vi "Lin Daten laden speichern.vi"(6 "Stufen Tabelle":T1, 9 "Lin Daten":T2 {"CalGas Eingang" items=["Cal Gas 1", "Cal Gas 2", "Cal Gas 3"]; "Max Fehler (Sollwert)" format="%#_5g"; "Zeitdauer Stufe" format="%#_5g"; "Anzahl Stufen" format="%#_5g"; "Verdünnungsgas" items=["N2", "O2"]}, 11 "Aktionen":T6) -> (0 "Stufen Tabellen":T1, 1 "Lin Daten Array":T2 {"CalGas Eingang" items=["Cal Gas 1", "Cal Gas 2", "Cal Gas 3"]; "Max Fehler (Sollwert)" format="%#_5g"; "Zeitdauer Stufe" format="%#_5g"; "Anzahl Stufen" format="%#_5g"; "Verdünnungsgas" items=["N2", "O2"]}, 3 "Gefunden?":bool)   [LabVIEW 2020, in "Linearisierung v2.lvlib" / "Gasteiler.lvlib"]
uses:
  Gasteiler.lvlib
  Lin Daten.ctl
  Visualisierungs Elemente/String - Eingabefeld.ctl
  Visualisierungs Elemente/Zahlen-Eingabefeld.ctl
  Lin Daten verwalten Aktionen.ctl
  Stufen Tabelle.ctl
  Seiten/FT-IR/FGV FT-IR Gasliste Aktionen.ctl
  Messdaten/Aktionen FGV Messdaten.ctl
  <vilib>/Utility/config.llb/Write Key (String).vi
  <vilib>/Utility/config.llb/Write Key (U32).vi
  <vilib>/Utility/config.llb/Write Key (Double).vi
  <vilib>/Utility/config.llb/Read Key (Double).vi
  <vilib>/Utility/config.llb/Read Key (U32).vi
  <vilib>/Utility/config.llb/Read Key (String).vi
  <vilib>/Utility/config.llb/NI_LVConfig.lvlib
  Allgemein/allgemeine Sub-VIs.lvlib
  Seiten/FT-IR/FT-IR.lvlib
  Messdaten/Messdaten.lvlib
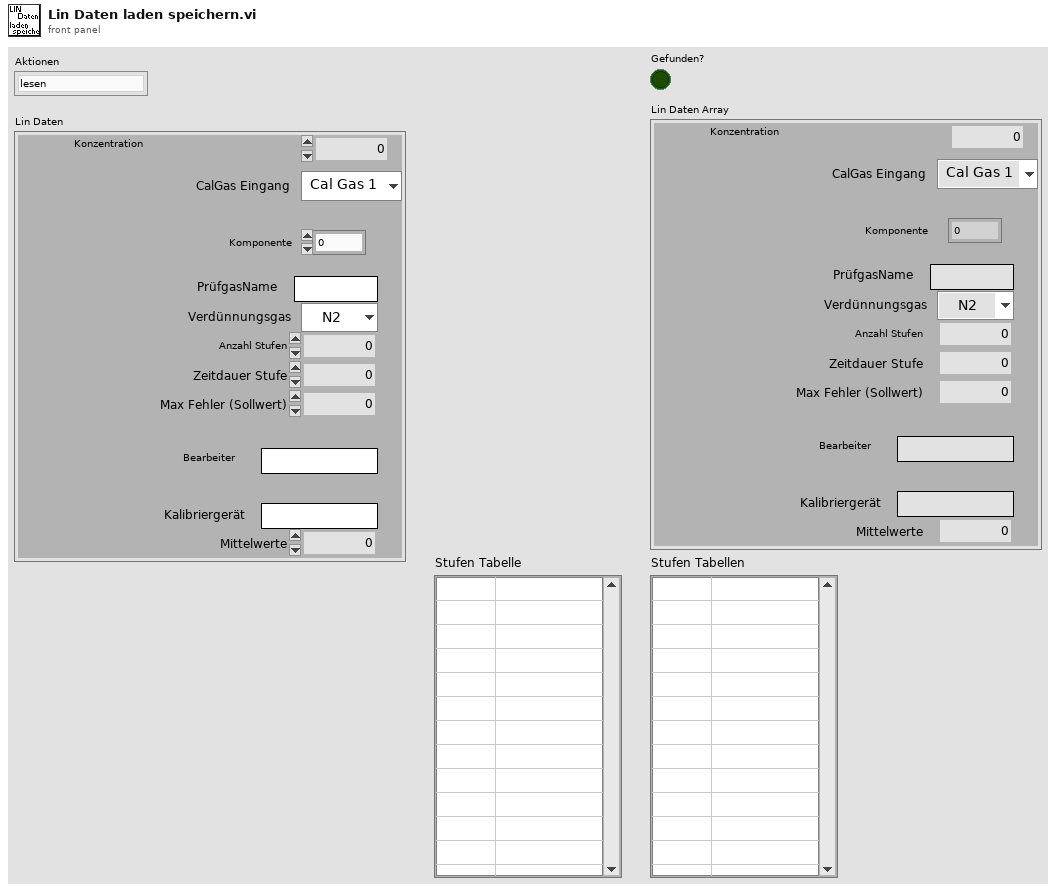
[diagram p1: front panel]
types:
  T1 = typedef "Linearisierung v2.lvlib/Gasteiler.lvlib/Stufen Tabelle.ctl" = string[][]
  T2 = typedef "Linearisierung v2.lvlib/Gasteiler.lvlib/Lin Daten.ctl" = cluster{"PrüfgasName":T3, "Verdünnungsgas":T4, "Anzahl Stufen":T5, "Zeitdauer Stufe":T5, "Max Fehler (Sollwert)":T5, "Bearbeiter":T3, "Kalibriergerät":T3, "Mittelwerte":i32, "Komponente":u16, "CalGas Eingang":u16, "Konzentration":sgl}
  T3 = typedef "String - Eingabefeld.ctl" = string
  T4 = typedef "Linearisierung v2.lvlib/Gasteiler.lvlib/Prüfgas in.ctl" = u16
  T5 = typedef "Zahlen-Eingabefeld.ctl" = sgl
  T6 = typedef "Linearisierung v2.lvlib/Gasteiler.lvlib/Lin Daten verwalten Aktionen.ctl" = enum16{"lesen", "speichern", "laden", "Lin Daten schr.", "Stufen Tabelle", "Lin Name AK", "Lin Pfad AK", "Umkehren"}
  T7 = typedef "Messdaten.lvlib/Aktionen FGV Messdaten.ctl" = enum16{"lesen", "schreiben", "löschen", "Mittelwerte", "Komponente"}
  T8 = typedef "FT-IR.lvlib/FGV FT-IR Gasliste Aktionen.ctl" = enum16{"lesen", "Gasliste FT-IR", "Gasliste ausgelesen", "laden", "speichern", "löschen"}
  T9 = typedef "String - Ausgabefeld.ctl" = string
  T10 = typedef "NI_LVConfig.lvlib/Config Data RefNum.ctl" = refnum<k1>
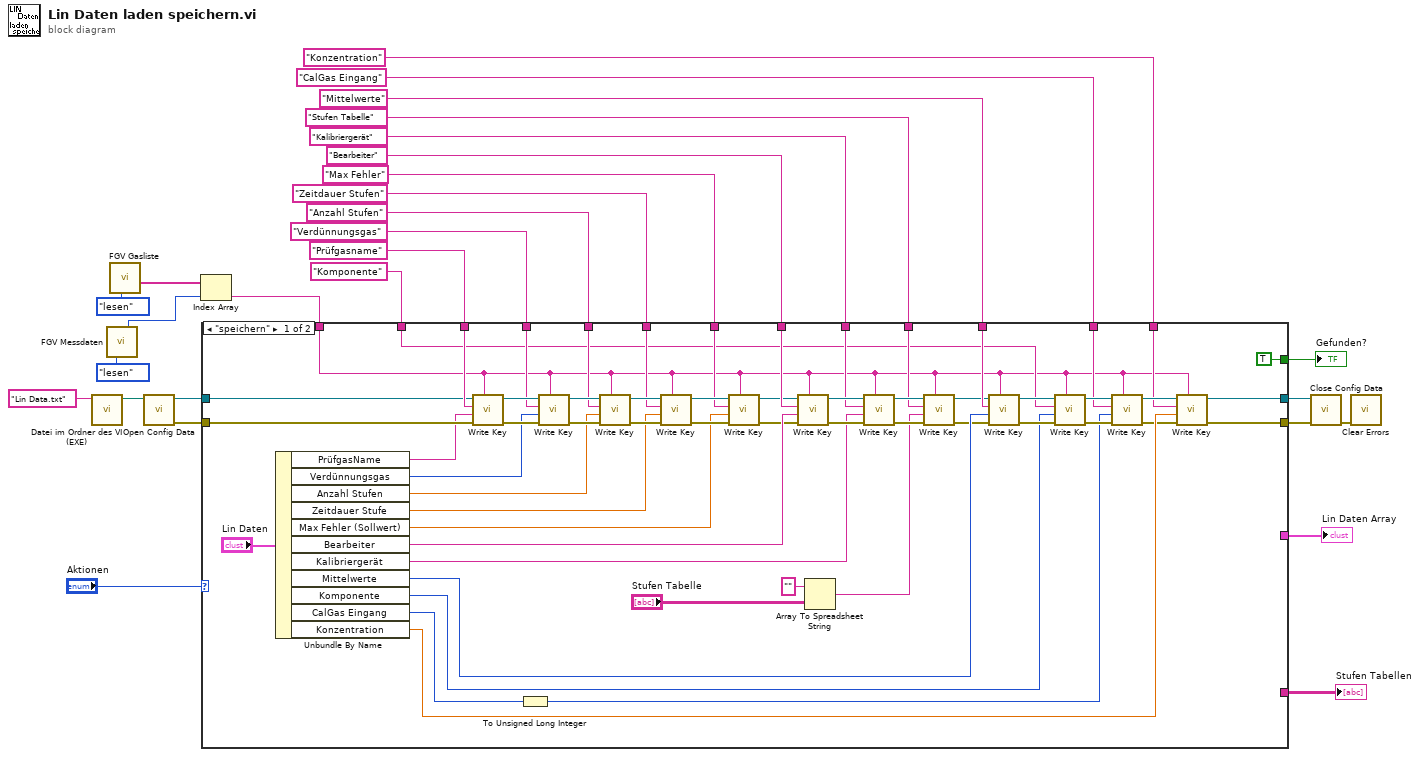
[diagram p0: block diagram]
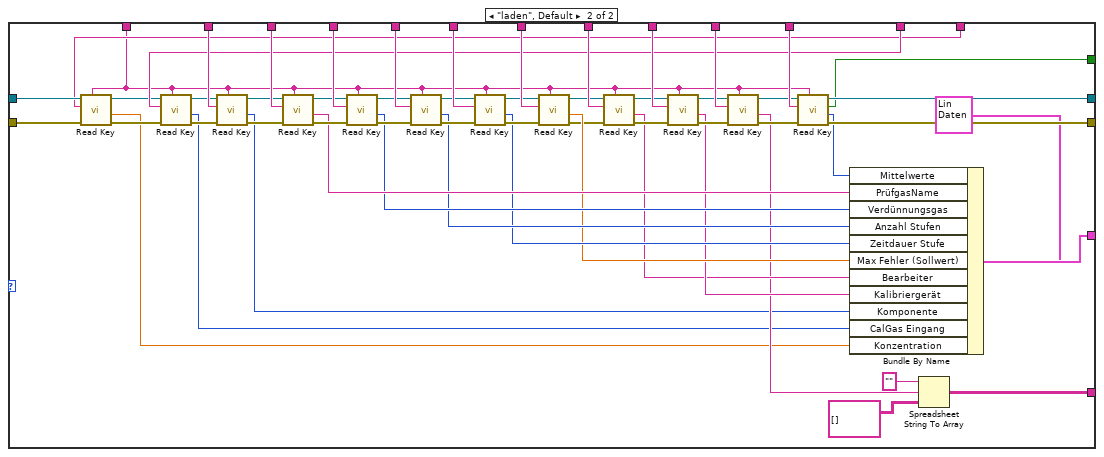
[diagram p2: hidden frame]
diagram:
  n1 = call "Datei im Ordner des VI (EXE).vi"("Dateiname"="Lin Data.txt") -> ("Dateipfad im Ordner des Haupt-VIs"=w28:path)  [unwired: 8 in, 2 out]
  n2 = call "FGV Messdaten.vi"("Aktionen"=Aktionen_FGV_Messdaten."lesen") -> ("Komponente"=w6:u16)  [unwired: 6 in, 8 out]
  n3 = call "FGV Gasliste.vi"("Aktionen"=FGV_FT-IR_Gasliste_Aktionen."lesen") -> ("Aktuelle Gasliste gesamt"=w4:T9[])  [unwired: 8 in, 2 out]
  n4 = call <vilib>:"Open Config Data.vi"("configuration file path"=w28) -> ("error out"=w25:errorcluster, "refnum"=w26:T10)  [unwired: 8 in, 1 out]
  n5 = Index Array(array=w4, index=w6) -> (element=w2:T9)
  n6 = case shown="\"speichern\"" "Aktionen" {
    tunnel: w26 -> [w52 w93]
    tunnel: w25 -> [w51 w92]
    tunnel: [w35 w141] -> w24
    tunnel: [w34 w140] -> w23
    tunnel: "Prüfgasname" ("key") -> [w69 w139]
    tunnel: "Verdünnungsgas" ("key") -> [w68 w138]
    tunnel: "Anzahl Stufen" ("key") -> [w67 w137]
    tunnel: "Zeitdauer Stufen" ("key") -> [w66 w136]
    tunnel: "Max Fehler" ("key") -> [w65 w135]
    tunnel: "Bearbeiter" ("key") -> [w64 w134]
    tunnel: "Kalibriergerät" ("key") -> [w63 w133]
    tunnel: "Stufen Tabelle" ("key") -> [w59 w132]
    tunnel: "Mittelwerte" ("key") -> [w54 w130]
    tunnel: [_ w131] -> w11
    tunnel: [_ w102] -> w10
    tunnel: "Komponente" ("key") -> [w44 w98]
    tunnel: "CalGas Eingang" ("key") -> [w40 w95]
    tunnel: "Konzentration" ("key") -> [w33 w89]
    tunnel: w2 -> [w30 w86]
    tunnel: [TRUE ("found?") w85] -> w1
    frame "speichern" {
      n7 = Unbundle By Name("Lin Daten") -> ("PrüfgasName"=w32:T3, "Verdünnungsgas"=w73:T4, "Anzahl Stufen"=w72:T5, "Zeitdauer Stufe"=w71:T5, "Max Fehler (Sollwert)"=w70:T5, "Bearbeiter"=w56:T3, "Kalibriergerät"=w55:T3, "Mittelwerte"=w53:i32, "Komponente"=w31:u16, "CalGas Eingang"=w41:u16, "Konzentration"=w38:sgl)
      n8 = call-poly <vilib>:"Write Key.vi"("section"=w30, "error in (no error)"=w51, "value"=w32, "key"=w69, "refnum"=w52) -> ("error out"=w84:errorcluster, "refnum out"=w83:T10)  [unwired: 4 in, 1 out]
      n9 = To Unsigned Long Integer(number=w41) -> (unsigned 32bit integer=w39:u32)
      n10 = call-poly <vilib>:"Write Key.vi"("section"=w30, "error in (no error)"=w84, "value"=w73, "key"=w68, "refnum"=w83) -> ("error out"=w82:errorcluster, "refnum out"=w81:T10)  [unwired: 4 in, 1 out]
      n11 = call-poly <vilib>:"Write Key.vi"("section"=w30, "error in (no error)"=w82, "value"=w72, "key"=w67, "refnum"=w81) -> ("error out"=w76:errorcluster, "refnum out"=w79:T10)  [unwired: 4 in, 1 out]
      n12 = call-poly <vilib>:"Write Key.vi"("section"=w30, "error in (no error)"=w76, "value"=w71, "key"=w66, "refnum"=w79) -> ("error out"=w75:errorcluster, "refnum out"=w78:T10)  [unwired: 4 in, 1 out]
      n13 = call-poly <vilib>:"Write Key.vi"("section"=w30, "error in (no error)"=w75, "value"=w70, "key"=w65, "refnum"=w78) -> ("error out"=w49:errorcluster, "refnum out"=w50:T10)  [unwired: 4 in, 1 out]
      n14 = call-poly <vilib>:"Write Key.vi"("section"=w30, "error in (no error)"=w49, "value"=w56, "key"=w64, "refnum"=w50) -> ("error out"=w74:errorcluster, "refnum out"=w77:T10)  [unwired: 4 in, 1 out]
      n15 = Array To Spreadsheet String(array="Stufen Tabelle", 3:"" ("Format-String")) -> (spreadsheet string=w58:string)  [unwired: 1 in]
      n16 = call-poly <vilib>:"Write Key.vi"("section"=w30, "error in (no error)"=w74, "value"=w55, "key"=w63, "refnum"=w77) -> ("error out"=w60:errorcluster, "refnum out"=w61:T10)  [unwired: 4 in, 1 out]
      n17 = call-poly <vilib>:"Write Key.vi"("section"=w30, "error in (no error)"=w60, "value"=w58, "key"=w59, "refnum"=w61) -> ("error out"=w47:errorcluster, "refnum out"=w48:T10)  [unwired: 4 in, 1 out]
      n18 = call-poly <vilib>:"Write Key.vi"("section"=w30, "error in (no error)"=w47, "value"=w53, "key"=w54, "refnum"=w48) -> ("error out"=w45:errorcluster, "refnum out"=w46:T10)  [unwired: 4 in, 1 out]
      n19 = call-poly <vilib>:"Write Key.vi"("section"=w30, "error in (no error)"=w45, "value"=w31, "key"=w44, "refnum"=w46) -> ("error out"=w43:errorcluster, "refnum out"=w42:T10)  [unwired: 4 in, 1 out]
      n20 = call-poly <vilib>:"Write Key.vi"("section"=w30, "error in (no error)"=w43, "value"=w39, "key"=w40, "refnum"=w42) -> ("error out"=w37:errorcluster, "refnum out"=w36:T10)  [unwired: 4 in, 1 out]
      n21 = call-poly <vilib>:"Write Key.vi"("section"=w30, "error in (no error)"=w37, "value"=w38, "key"=w33, "refnum"=w36) -> ("error out"=w34:errorcluster, "refnum out"=w35:T10)  [unwired: 4 in, 1 out]
    }
    frame "laden", Default {
      n22 = call-poly <vilib>:"Read Key.vi"("section"=w86, "error in (no error)"=w92, "key"=w89, "refnum"=w93) -> ("error out"=w91:errorcluster, "value"=w88:dbl, "refnum out"=w90:T10)  [unwired: 4 in, 1 out]
      n23 = call-poly <vilib>:"Read Key.vi"("section"=w86, "error in (no error)"=w91, "key"=w95, "refnum"=w90) -> ("error out"=w96:errorcluster, "value"=w94:u32, "refnum out"=w97:T10)  [unwired: 4 in, 1 out]
      n24 = call-poly <vilib>:"Read Key.vi"("section"=w86, "error in (no error)"=w96, "key"=w98, "refnum"=w97) -> ("error out"=w99:errorcluster, "value"=w87:u32, "refnum out"=w100:T10)  [unwired: 4 in, 1 out]
      n25 = call-poly <vilib>:"Read Key.vi"("section"=w86, "error in (no error)"=w99, "key"=w139, "refnum"=w100) -> ("error out"=w128:errorcluster, "value"=w118:string, "refnum out"=w129:T10)  [unwired: 4 in, 1 out]
      n26 = call-poly <vilib>:"Read Key.vi"("section"=w86, "error in (no error)"=w128, "key"=w138, "refnum"=w129) -> ("error out"=w126:errorcluster, "value"=w117:u32, "refnum out"=w127:T10)  [unwired: 4 in, 1 out]
      n27 = call-poly <vilib>:"Read Key.vi"("section"=w86, "error in (no error)"=w126, "key"=w137, "refnum"=w127) -> ("error out"=w124:errorcluster, "value"=w116:u32, "refnum out"=w125:T10)  [unwired: 4 in, 1 out]
      n28 = call-poly <vilib>:"Read Key.vi"("section"=w86, "error in (no error)"=w124, "key"=w136, "refnum"=w125) -> ("error out"=w122:errorcluster, "value"=w115:u32, "refnum out"=w123:T10)  [unwired: 4 in, 1 out]
      n29 = call-poly <vilib>:"Read Key.vi"("section"=w86, "error in (no error)"=w122, "key"=w135, "refnum"=w123) -> ("error out"=w107:errorcluster, "value"=w114:dbl, "refnum out"=w108:T10)  [unwired: 4 in, 1 out]
      n30 = call-poly <vilib>:"Read Key.vi"("section"=w86, "error in (no error)"=w107, "key"=w134, "refnum"=w108) -> ("error out"=w120:errorcluster, "value"=w110:string, "refnum out"=w121:T10)  [unwired: 4 in, 1 out]
      n31 = call-poly <vilib>:"Read Key.vi"("section"=w86, "error in (no error)"=w120, "key"=w133, "refnum"=w121) -> ("error out"=w113:errorcluster, "value"=w111:string, "refnum out"=w112:T10)  [unwired: 4 in, 1 out]
      n32 = call-poly <vilib>:"Read Key.vi"("section"=w86, "error in (no error)"=w113, "key"=w132, "refnum"=w112) -> ("error out"=w105:errorcluster, "value"=w104:string, "refnum out"=w106:T10)  [unwired: 4 in, 1 out]
      n33 = call-poly <vilib>:"Read Key.vi"("section"=w86, "error in (no error)"=w105, "key"=w130, "refnum"=w106) -> ("error out"=w140:errorcluster, "value"=w109:u32, "found?"=w85:bool, "refnum out"=w141:T10)  [unwired: 4 in]
      n34 = Bundle By Name(cluster=T2 {"PrüfgasName"="", "Verdünnungsgas"=0, "Anzahl Stufen"=0.0, "Zeitdauer Stufe"=0.0, "Max Fehler (Sollwert)"=0.0, "Bearbeiter"="", "Kalibriergerät"="", "Mittelwerte"=0, "Komponente"=0, "CalGas Eingang"=0, "Konzentration"=0.0} ("Lin Daten"), "Mittelwerte"=w109, "PrüfgasName"=w118, "Verdünnungsgas"=w117, "Anzahl Stufen"=w116, "Zeitdauer Stufe"=w115, "Max Fehler (Sollwert)"=w114, "Bearbeiter"=w110, "Kalibriergerät"=w111, "Komponente"=w87, "CalGas Eingang"=w94, "Konzentration"=w88) -> (w131:T2)
      n35 = Spreadsheet String To Array(format string="" ("Format-String"), spreadsheet string=w104, array type (2D Dbl)=T1 [] ("Stufen Tabelle")) -> (array=w102:string[][])  [unwired: 1 in]
    }
  }
  "Lin Daten Array" <- w11
  "Stufen Tabellen" <- w10
  "Gefunden?" <- w1
  n36 = call <vilib>:"Close Config Data.vi"("error in (no error)"=w23, "refnum"=w24) -> ("error out"=w14:errorcluster)  [unwired: 8 in, 1 out]
  n37 = call <vilib>:"Clear Errors.vi"("error in (no error)"=w14) -> ()  [unwired: 5 in, 2 out]
